vi "Detectors Crl_AE.vi"(7 "Action":enum16{"READ", "WRITE"}(ring), 10 "Detectors Parameters In":T1) -> (2 "Detectors Parameters Out":T1)   [LabVIEW 2014]
uses:
  Host VIs/Detectors.ctl
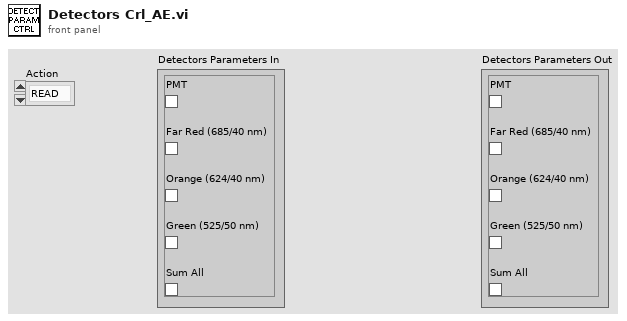
[diagram p1: front panel]
types:
  T1 = typedef "Detectors.ctl" = cluster{"PMT":bool, "Far Red (685/40 nm)":bool, "Orange (624/40 nm)":bool, "Green (525/50 nm)":bool, "Sum All":bool}
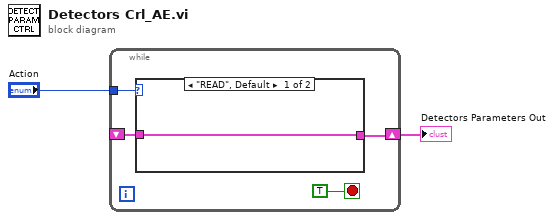
[diagram p0: block diagram]
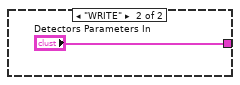
[diagram p2: hidden frame]
diagram:
  n1 = while {
    tunnel: "Action" -> [w5]
    shift-right: [w4] -> w1
    shift-left: _ -> [w3]
    stop <- TRUE stop-if-true
    n2 = case shown="\"READ\", Default" w5 {
      tunnel: [w7 "Detectors Parameters In"] -> w4
      tunnel: w3 -> [w7 _]
      frame "READ", Default {
      }
      frame "WRITE" {
      }
    }
  }
  "Detectors Parameters Out" <- w1
